vi "State.gbl.vi"() -> ()   [LabVIEW 2020, in "NI_PID__autopid compat.lvlib"]
doc: "This global is used to track the state of the autotuning procedure."
uses:
  <vilib>/addons/control/pid/NI_PID__autopid compat.lvlib
panel:
  in  "current state":T1(ring)=enum."Start"
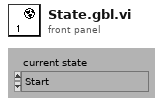
[diagram p1: front panel]
types:
  T1 = enum16{"Normal", "Start", "Check params", "Check noise", "Start noise est.", "Re-estimate noise", "Begin autotune", "Autotuning", "New parameters", ""}
diagram:
